vi "MT Align to Ideal Symbols (Generic).vi"(0 "input complex waveform":T1={"t0"=0.0, "dt"=1.0, "Y"=[]} {"Y" format="%.3f"; "dt" format="%^.2e"; "t0" format="%.4f"}, 5 "matched filter coefficients":dbl[](array[numeric]) format="%^.2e", 7 "samples per symbol (16)":i32=16, 11 "error in (no error)":errorcluster, 13 "reset? (T)":bool=TRUE) -> (4 "output complex waveform":T1 {"Y" format="%.3f"; "dt" format="%^.2e"; "t0" format="%.4f"}, 8 "waveform alignment offset (samples)":dbl, 15 "error out":errorcluster)   [LabVIEW 2020, in "niDMT.lvlib"]
doc: "This polymorphic instance aligns the first sample of the <B>input complex waveform</B> to the ideal symbol timing instant for PAM, ASK, QAM, and nonoffset PSK modulation schemes."
uses:
  <vilib>/addons/Modulation/niDMT.lvlib
  <vilib>/addons/Modulation/Analog/controls/Complex Data Waveform.ctl
  <vilib>/addons/Modulation/niAMT.lvlib
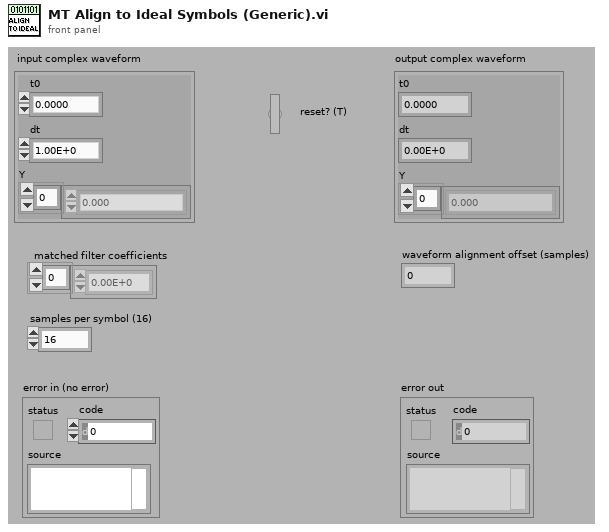
[diagram p1: front panel]
types:
  T1 = typedef "niAMT.lvlib/Complex Data Waveform.ctl" = cluster{"t0":dbl, "dt":dbl, "Y":cdb[]}
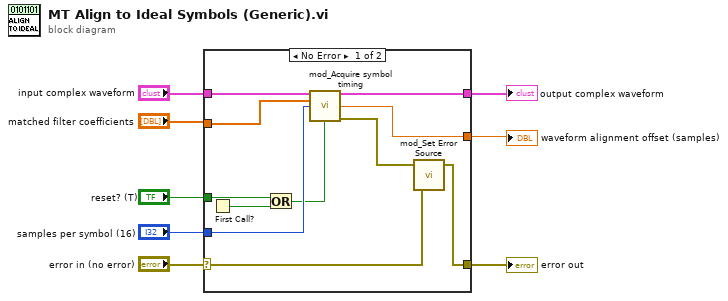
[diagram p0: block diagram]
diagram:
  n1 = case shown="No Error" "error in (no error)" {
    selector: "error in (no error)" -> [w9 w20]
    tunnel: "input complex waveform" -> [w19 _]
    tunnel: "matched filter coefficients" -> [w18 _]
    tunnel: "samples per symbol (16)" -> [w13 _]
    tunnel: "reset? (T)" -> [w17 _]
    tunnel: [w14 _] -> w3
    tunnel: [w15 _] -> w2
    tunnel: [w10 w20] -> w1
    frame No Error {
      n2 = First Call?() -> (First Call?: T/F=w16:bool)
      n3 = Or(x=w17, y=w16) -> (x .or. y?=w12:bool)
      n4 = call <vilib>:"mod_Acquire symbol timing.vi"("input complex waveform"=w19, "matched filter coefficients"=w18, "samples per symbol (16)"=w13, "reset? (T)"=w12) -> ("output complex waveform"=w14:T1, "waveform alignment offset"=w15:dbl, "error out"=w11:errorcluster)  [unwired: 1 in, 8 out]
      n5 = call <vilib>:"mod_Set Error Source.vi"("initial error in (no error)"=w9, "final error in (no error)"=w11) -> ("error out"=w10:errorcluster)  [unwired: 3 out]
    }
    frame Error {
    }
  }
  "error out" <- w1
  "output complex waveform" <- w3
  "waveform alignment offset (samples)" <- w2
